vi "PanelBoundsToDesciptiveString.vi"(8 "error in (no error)":errorcluster, 10 "Panel Bounds":T1) -> (0 "error out":errorcluster, 3 "String":string)   [LabVIEW 2023]
uses:
  <vilib>/Utility/miscctls.llb/LVRectTypeDef.ctl
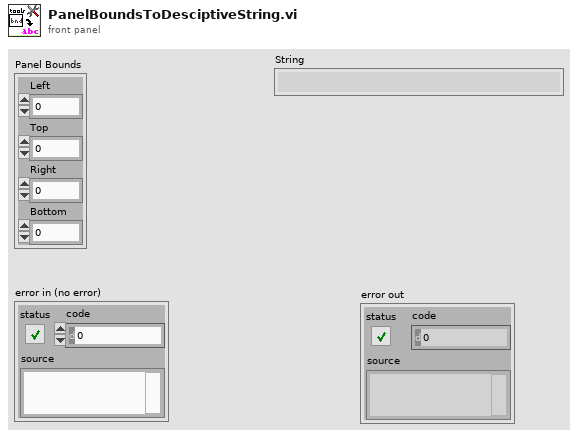
[diagram p1: front panel]
types:
  T1 = typedef "LVRectTypeDef.ctl" = cluster{"Left":i16, "Top":i16, "Right":i16, "Bottom":i16}
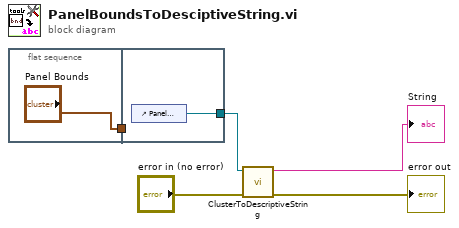
[diagram p0: block diagram]
diagram:
  n1 = flat-sequence {
    tunnel: ["Panel Bounds"] -> w1
    tunnel: [w7] -> w3
    tunnel: w1 -> [_]
    frame #0 {
    }
    frame #1 {
      n2 = control-ref of="Panel Bounds"() -> (w7:refnum<vi>)
    }
  }
  n3 = call "ClusterToDescriptiveString.vi"("error in"="error in (no error)", "Cluster In"=w3) -> ("error out"=→"error out":errorcluster, "String"=→"String":string)  [unwired: 8 in]
